vi "BEGIN.vi"(7 "Savepoint name":string, 8 "error in (no error)":errorcluster, 11 "Connection in":refnum<class "Connection.lvclass">) -> (0 "error out":errorcluster, 3 "Connection out":refnum<class "Connection.lvclass">)   [LabVIEW 2013, in "SQLiteSupport.lvlib" / "Transaction.lvlib"]
doc: "Start a transaction using \"BEGIN IMMEDIATE\". \n\nIf an optional Savepoint name is provided then a SAVEPOINT is created. Savepoints can be nested.\n\nNote that open transactions maintain an exclusive write-lock on the database file. See SQLite.org documentation."
uses:
  Transaction.lvlib
  SQL Connection/Connection.lvclass
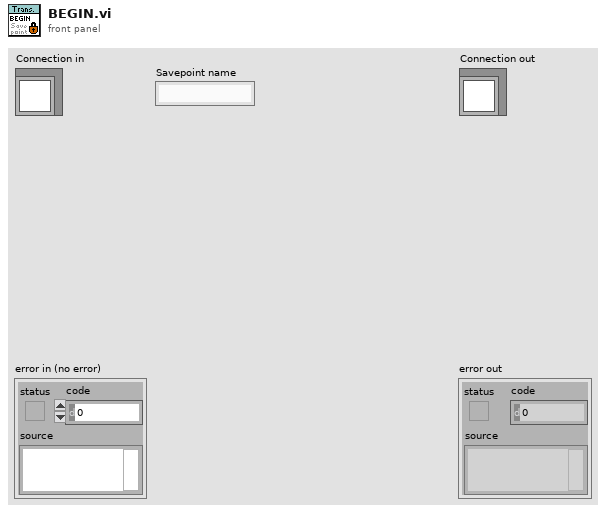
[diagram p1: front panel]
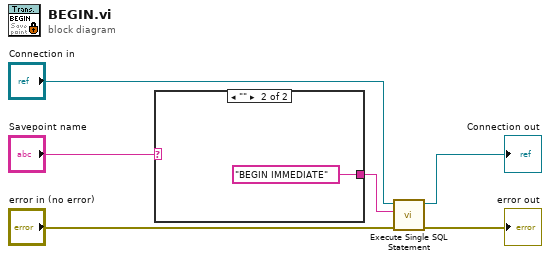
[diagram p0: block diagram]
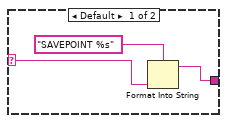
[diagram p2: hidden frame]
diagram:
  n1 = case shown="\"\"" "Savepoint name" {
    selector: "Savepoint name" -> [w9 _]
    tunnel: [w7 "BEGIN IMMEDIATE"] -> w1
    frame Default {
      n2 = Format Into String(format string="SAVEPOINT %s", w9) -> (resulting string=w7:string)  [unwired: 2 in, 1 out]
    }
    frame "" {
    }
  }
  n3 = call "Execute Single SQL Statement.vi"("error in (no error)"="error in (no error)", "SQL statement"=w1, "SQLite Connection in"="Connection in") -> ("error out"=→"error out":errorcluster, "SQLite Connection out"=→"Connection out":refnum<class "Connection.lvclass">)  [unwired: 7 in]
